vi "ReadRoughGainandFineGain.vi"(8 "error in (no error)":errorcluster, 10 "reference":refnum<k7>, 11 "IN":T1={"step name 1"="", "updata 2"="1000", "limitdata 3"="", "load vi name 4"="", "parameter 5"=""}) -> (0 "error out":errorcluster, 2 "reference out":refnum<k7>, 3 "Cluster":T2)   [LabVIEW 2013]
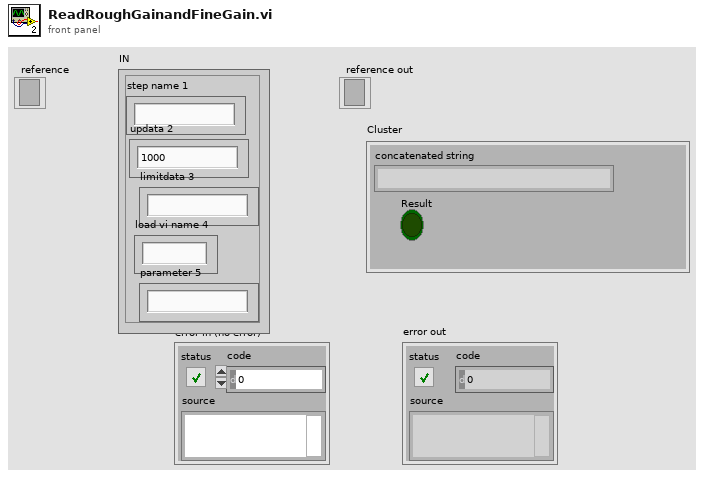
[diagram p1: front panel]
types:
  T1 = cluster{"step name 1":string, "updata 2":string, "limitdata 3":string, "load vi name 4":string, "parameter 5":string}
  T2 = cluster{"concatenated string":string, "Result":bool}
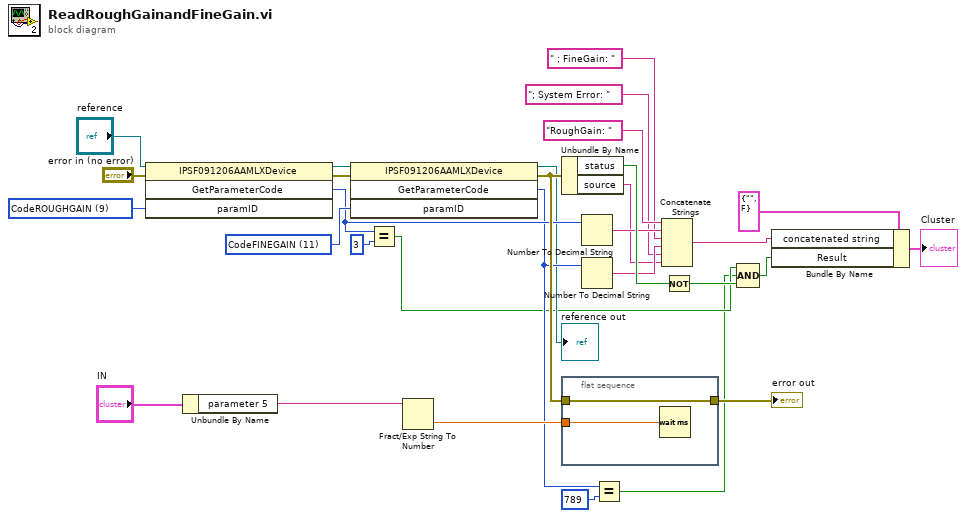
[diagram p0: block diagram]
diagram:
  w20 = 11 items=["CodeTC2ND"=1, "CodeTC1ST"=2, "CodeOFFDRIFT"=3, "CodeFILTCODE"=4, "CodeDCDEF"=5, "CodeSWITCH"=6, "CodeCLAMP"=7, "CodeOUTMODE"=8, "CodeROUGHGAIN"=9, "CodeOUTSLOPE"=10, "CodeFINEGAIN"=11, "CodeDIAGINFAULT"=12, "CodeREFEDGE"=13, "CodeYA"=14, "CodeXA"=15, "CodeCSTID"=16, "CodeMLXID1"=17, "CodeMLXID2"=18, "CodeMLXID3"=19, "CodeCRC10"=20, "CodeRATIODIS"=21, "CodeTC2NDHOT"=22, "CodeTC2NDCOLD"=23, "CodeOFFDRIFTHOT"=24, "CodeOFFDRIFTCOLD"=25, "CodeCLAMPLOW"=26, "CodeCLAMPHIGH"=27, "CodePLATEPOL"=28, "CodeDSPMODE"=104, "CodeTHERMOSLOPE"=106, "CodeTHERMOOFF"=107, "CodeDeltaTC1ST_RGP1"=29, "CodeDeltaTC1ST_RGM1"=30, "CodeDeltaOD_RGP1"=31, "CodeDeltaOD_RGM1"=32, "CodeOPTIONCODE"=33, "CodeLOTNUMBER"=34] ("paramID")
  w24 = 9 items=["CodeTC2ND"=1, "CodeTC1ST"=2, "CodeOFFDRIFT"=3, "CodeFILTCODE"=4, "CodeDCDEF"=5, "CodeSWITCH"=6, "CodeCLAMP"=7, "CodeOUTMODE"=8, "CodeROUGHGAIN"=9, "CodeOUTSLOPE"=10, "CodeFINEGAIN"=11, "CodeDIAGINFAULT"=12, "CodeREFEDGE"=13, "CodeYA"=14, "CodeXA"=15, "CodeCSTID"=16, "CodeMLXID1"=17, "CodeMLXID2"=18, "CodeMLXID3"=19, "CodeCRC10"=20, "CodeRATIODIS"=21, "CodeTC2NDHOT"=22, "CodeTC2NDCOLD"=23, "CodeOFFDRIFTHOT"=24, "CodeOFFDRIFTCOLD"=25, "CodeCLAMPLOW"=26, "CodeCLAMPHIGH"=27, "CodePLATEPOL"=28, "CodeDSPMODE"=104, "CodeTHERMOSLOPE"=106, "CodeTHERMOOFF"=107, "CodeDeltaTC1ST_RGP1"=29, "CodeDeltaTC1ST_RGM1"=30, "CodeDeltaOD_RGP1"=31, "CodeDeltaOD_RGM1"=32, "CodeOPTIONCODE"=33, "CodeLOTNUMBER"=34] ("paramID")
  n1 = invoke class="IPSF091206AAMLXDevice" method="GetParameterCode"(reference="reference", error in="error in (no error)", "paramID"=w24) -> (reference out=w23:refnum<k7>, error out=w22:errorcluster, "GetParameterCode"=w12:i32)  [unwired: 1 in, 1 out]
  n2 = Unbundle By Name("IN") -> ("parameter 5"=w26:string)
  n3 = invoke class="IPSF091206AAMLXDevice" method="GetParameterCode"(reference=w23, error in=w22, "paramID"=w20) -> (reference out=→"reference out":refnum<k7>, error out=w17:errorcluster, "GetParameterCode"=w10:i32)  [unwired: 1 in, 1 out]
  n4 = Equal?(x=w12, y=3) -> (x = y?=w2:bool)
  n5 = Fract/Exp String To Number(string=w26) -> (number=w27:dbl)  [unwired: 3 in, 1 out]
  n6 = Unbundle By Name(w17) -> ("status"=w16:bool, "source"=w6:string)
  n7 = flat-sequence {
    tunnel: w27 -> [w32]
    tunnel: [w31] -> w21
    tunnel: w17 -> [w31]
    frame #0 {
      n8 = Wait (ms)(milliseconds to wait=w32) -> ()  [unwired: 1 out]
    }
  }
  n9 = Number To Decimal String(number=w12) -> (decimal integer string=w11:string)  [unwired: 1 in]
  n10 = Number To Decimal String(number=w10) -> (decimal integer string=w8:string)  [unwired: 1 in]
  n11 = Equal?(x=w10, y=789) -> (x = y?=w1:bool)
  n12 = Concatenate Strings("RoughGain: " ("string"), w11, " ; FineGain: " ("string"), w8, "; System Error: " ("string"), w6) -> (w5:string)
  n13 = Not(x=w16) -> (.not. x?=w15:bool)
  n14 = Compound Arithmetic op=AND(w2, w1, w15) -> (w14:bool)
  n15 = Bundle By Name(cluster=T2 {"concatenated string"="", "Result"=FALSE} ("Cluster"), "concatenated string"=w5, "Result"=w14) -> (→"Cluster":T2)
  "error out" <- w21
